vi "Initialize.vi"(11 "data in":refnum<class "EventMessengerPData.lvclass">) -> (1 "Event Registration Refnum":refnum<event-registration>, 3 "data out":refnum<class "EventMessengerPData.lvclass">)   [LabVIEW 2020, in "Event Messenger Priority.lvlib" / "EventMessengerPData.lvclass"]
uses:
  EventMessengerPData.lvclass
  EventMessengerPData.lvclass/EventMessengerPData.ctl
  Event Data.ctl
  Event Messenger Priority.lvlib
  Element.ctl
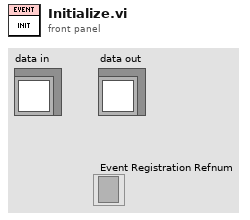
[diagram p1: front panel]
types:
  T1 = typedef "Event Messenger Priority.lvlib/Event Data.ctl" = cluster{"elt":T2, "elt valid?":bool, "last elt?":bool, "aborted?":bool, "priority?":bool}
  T2 = typedef "Event Messenger Priority.lvlib/Element.ctl" = cluster{"cmd":string, "data":variant}
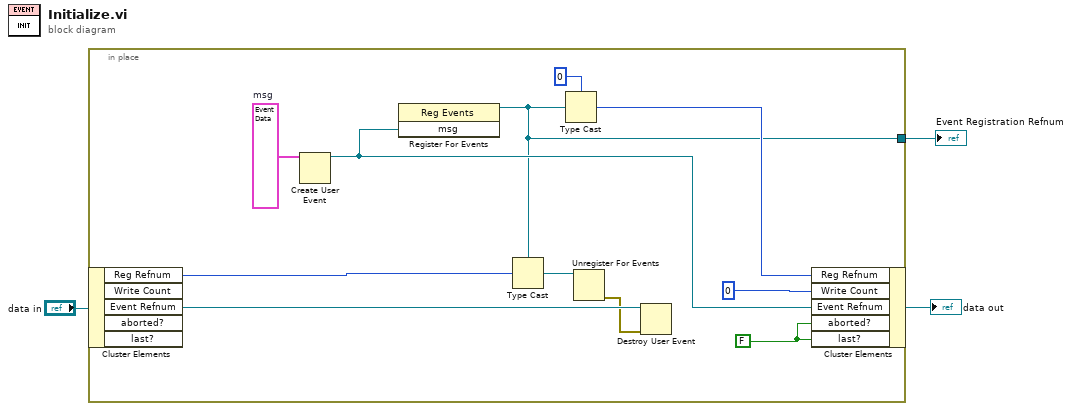
[diagram p0: block diagram]
diagram:
  n1 = in-place {
    in-place-border: [w5] -> w1
    w4 = T1 {"elt"={"cmd"="", "data"=variant}, "elt valid?"=TRUE, "last elt?"=TRUE, "aborted?"=TRUE, "priority?"=TRUE}  # msg
    w6 = FALSE ("aborted?")
    n2 = in-place-cluster #1("data in") -> ("Reg Refnum"=w14:u32, "Event Refnum"=w12:refnum<user-event>)  [unwired: 3 out]
    n3 = Create User Event(user event datatype=w4) -> (user event=w8:refnum<user-event>)  [unwired: 1 in, 1 out]
    n4 = register-events(w8) -> (reference out=w5:refnum<event-registration>)  [unwired: 2 in, 1 out]
    n5 = Type Cast(type=w5, x=w14) -> (*(type *) &x=w13:refnum<event-registration>)
    n6 = Type Cast(type=u32 0 ("Reg Refnum"), x=w5) -> (*(type *) &x=w7:u32)
    n7 = Unregister For Events(event registration refnum=w13) -> (error out=w11:errorcluster)  [unwired: 1 in]
    n8 = Destroy User Event(user event=w12, error in=w11) -> ()  [unwired: 1 out]
    n9 = in-place-cluster #1("Reg Refnum"=w7, "Write Count"=u32 0 ("Registration Count"), "Event Refnum"=w8, "aborted?"=w6, "last?"=w6) -> (→"data out":refnum<class "EventMessengerPData.lvclass">)
  }
  "Event Registration Refnum" <- w1
